vi "DtOLCloseTask.vi"(8 "Error in":errorcluster, 11 "Task in":i32) -> (0 "Error Out":errorcluster)   [LabVIEW 2022 SP3]
uses:
  DtLvLink.lvlib
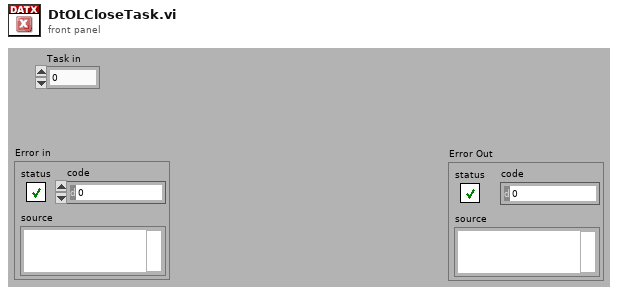
[diagram p1: front panel]
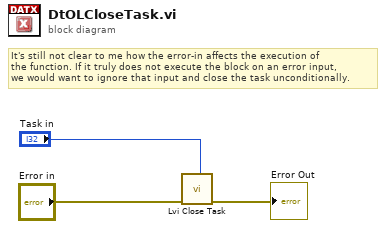
[diagram p0: block diagram]
diagram:
  # "It's still not clear to me how the error-in affects the execution of\nthe function. If it truly does not execute the block on an error input, \nwe would want to ignore that input and close the task unconditionally."
  n1 = call "Lvi Close Task.vi"("error in (no error)"="Error in", "TaskRef"="Task in") -> ("error out"=→"Error Out":errorcluster)  [unwired: 8 in, 1 out]
